vi "Debug String Helper.vi"(10 "error to print":errorcluster, 11 "Title":string) -> (0 "error out":errorcluster)   [LabVIEW 2020, in "afdx_custom_device Engine.lvlib"]
uses:
  afdx_custom_device Engine.lvlib
  <vilib>/NI_Real-Time Target Support.lvlib
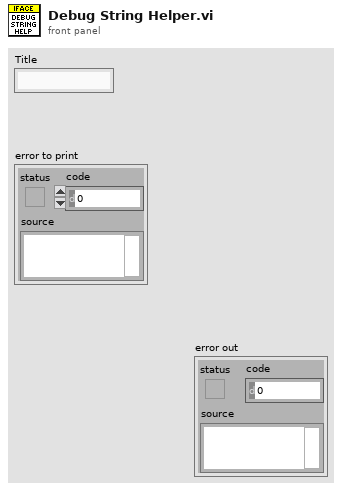
[diagram p1: front panel]
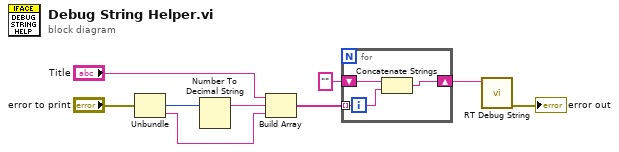
[diagram p0: block diagram]
diagram:
  n1 = Unbundle("error to print") -> ("code"=w4:i32, "source"=w5:string)  [unwired: 1 out]
  n2 = Number To Decimal String(number=w4) -> (decimal integer string=w3:string)  [unwired: 1 in]
  n3 = Build Array("Title", w3, w5) -> (w1:string[])
  n4 = for {
    shift-right: [w11] -> w8
    shift-left: "" -> [w12]
    tunnel: w1 -> [w10] mode=indexing
    n5 = Concatenate Strings(w12, w10) -> (w11:string)
  }
  n6 = call <vilib>:"RT Debug String.vi"("String to write"=w8) -> ("error out"=→"error out":errorcluster)  [unwired: 10 in]
